vi "matrici_v0_v45.vi"() -> ()   [LabVIEW 2009]
uses:
  <vilib>/Native 3D Graph/xcontrol/3DPC_SurfacePlot.xctl
panel:
  in  "Domeniul de definitie y":dbl(slide)=3.545075125208681 scale=-2.0..2.0
  out "3D Graph":refnum<class "Base Datatype.lvclass">[](xcontrol)
  out "X":dbl=1.7725375626043396
  in  "stop":bool
  in  "Domeniul de definitie x,y":dbl(slide)=3.545075125208681 scale=0.5..10.0
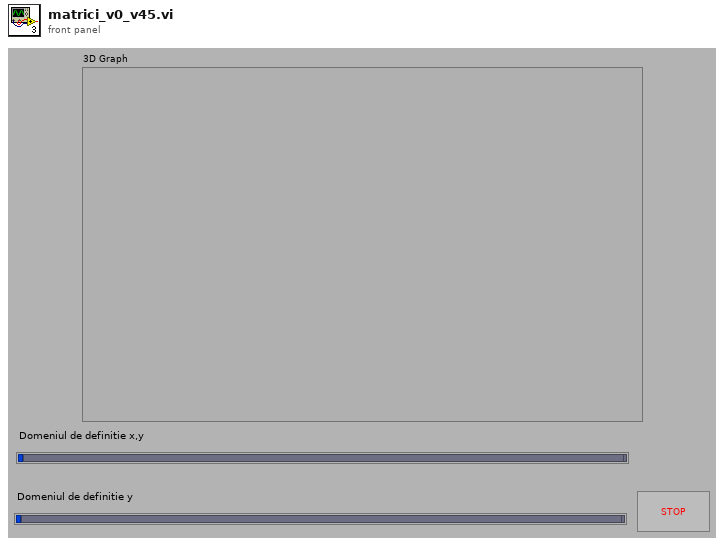
[diagram p1: front panel]
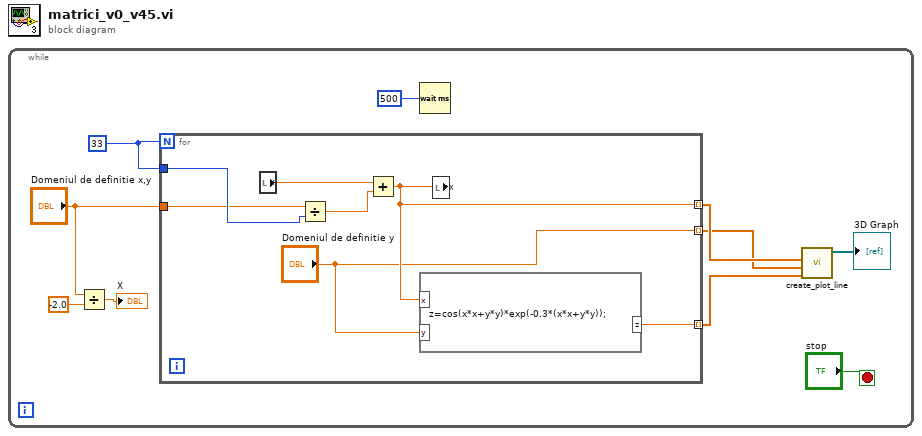
[diagram p0: block diagram]
diagram:
  n1 = while {
    stop <- "stop" stop-if-true
    w8 = 33
    n2 = Divide(x="Domeniul de definitie x,y", y=-2.0) -> (x/y=→"X":dbl)
    n3 = for {
      N: w8 -> [_]
      tunnel: [w13] -> w3 mode=indexing
      tunnel: w8 -> [w16]
      tunnel: "Domeniul de definitie x,y" -> [w15]
      tunnel: [w12] -> w1 mode=indexing
      tunnel: ["Domeniul de definitie y"] -> w2 mode=indexing
      n4 = local read "X"() -> (w17:dbl)
      n5 = Divide(x=w15, y=w16) -> (x/y=w14:dbl)
      n6 = Add(x=w17, y=w14) -> (x+y=w13:dbl)
      n7 = formula code="z=cos(x*x+y*y)*exp(-0.3*(x*x+y*y));"("x"=w13, "y"="Domeniul de definitie y") -> ("z"=w12:dbl)
      n8 = local write "X"(w13) -> ()
    }
    n9 = Wait (ms)(milliseconds to wait=500) -> ()  [unwired: 1 out]
    n10 = call <vilib>:"create_plot_line.vi"("z vector"=w1, "y vector"=w2, "x vector"=w3) -> ("plots out"=→"3D Graph":refnum<class "Base Datatype.lvclass">[])  [unwired: 2 in, 6 out]
  }
